vi "convertCSVDateToTimestamp.vi"(11 "date string":string) -> (3 "time stamp":timestamp)   [LabVIEW 2018]
uses:
  <vilib>/Utility/miscctls.llb/LVDateTimeRec.ctl
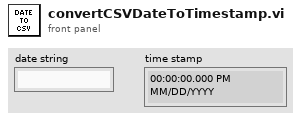
[diagram p1: front panel]
types:
  T1 = typedef "LVDateTimeRec.ctl" = cluster{"fractional second":dbl, "second":i32, "minute":i32, "hour":i32, "day of month":i32, "month":i32, "year":i32, "day of week":i32, "day of year":i32, "DST":i32}
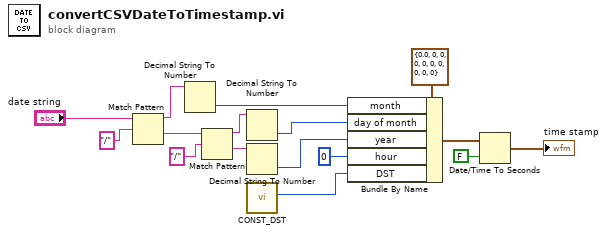
[diagram p0: block diagram]
diagram:
  n1 = Match Pattern(string="date string", regular expression="/") -> (before substring=w5:string, after substring=w7:string)  [unwired: 3 out]
  n2 = Decimal String To Number(string=w5) -> (number=w8:i32)  [unwired: 2 in, 1 out]
  n3 = Match Pattern(string=w7, regular expression="/") -> (before substring=w9:string, after substring=w11:string)  [unwired: 3 out]
  n4 = Decimal String To Number(string=w9) -> (number=w10:i32)  [unwired: 2 in, 1 out]
  n5 = Decimal String To Number(string=w11) -> (number=w12:i32)  [unwired: 2 in, 1 out]
  n6 = call "CONST_DST.vi"() -> ("DST"=w15:i32)  [unwired: 11 in]
  n7 = Bundle By Name(cluster=T1 {"fractional second"=0.0, "second"=0, "minute"=0, "hour"=0, "day of month"=0, "month"=0, "year"=0, "day of week"=0, "day of year"=0, "DST"=0} ("date time rec"), "month"=w8, "day of month"=w10, "year"=w12, "hour"=0 ("DST"), "DST"=w15) -> (w3:T1)
  n8 = Date/Time To Seconds(1:FALSE ("is UTC (F)"), 2:w3) -> (0:→"time stamp":timestamp)
